vi "Begin.vi"(11 "Image Size":T1=enum."160x120") -> (0 "error out":errorcluster)   [LabVIEW 2011]
doc: "Called before other user functions, this VI is expected to open initial I/O refnums, load in file data, and do all program initialization. Notice that the <B>error out</B> terminal is simply used for data flow. Wiring it to other structures or subVIs ensures that this VI runs first."
uses:
  <vilib>/Rock Robotics/WPI/Camera/WPI_CameraImageSize.ctl
  <vilib>/Rock Robotics/WPI/Joystick/WPI_JoystickDeviceEnum.ctl
  <vilib>/Rock Robotics/WPI/Camera/WPI_CameraWhite Balance Values.ctl
  <vilib>/Rock Robotics/WPI/Camera/WPI_CameraExposure Values.ctl
  <vilib>/Rock Robotics/WPI/Camera/WPI_CameraFrameRate.ctl
  <vilib>/Rock Robotics/SystemInterfaces/DIO/FPGA_DIOPWMChannel.ctl
  <vilib>/Rock Robotics/WPI/Relay/WPI_RelayDirection.ctl
  <vilib>/Rock Robotics/SystemInterfaces/DIO/FPGA_DIORelayChannel.ctl
  <vilib>/Rock Robotics/SystemInterfaces/Typedef/FPGA_TypedefDigitalModule.ctl
  <vilib>/Rock Robotics/SystemInterfaces/DIO/FPGA_DIOChannel.ctl
  <vilib>/Rock Robotics/WPI/Solenoid/WPI_SolenoidChannel.ctl
  <vilib>/Rock Robotics/WPI/MotorControl/WPI_MotorControlOpen Jaguar.vi
  <vilib>/Rock Robotics/WPI/MotorControl/WPI_MotorControlOpen Victor.vi
  <vilib>/Rock Robotics/WPI/RobotDrive/WPI_RobotDriveOpen4MotorWithJaguar.vi
  <vilib>/Rock Robotics/WPI/Solenoid/WPI_SolenoidOpenDouble.vi
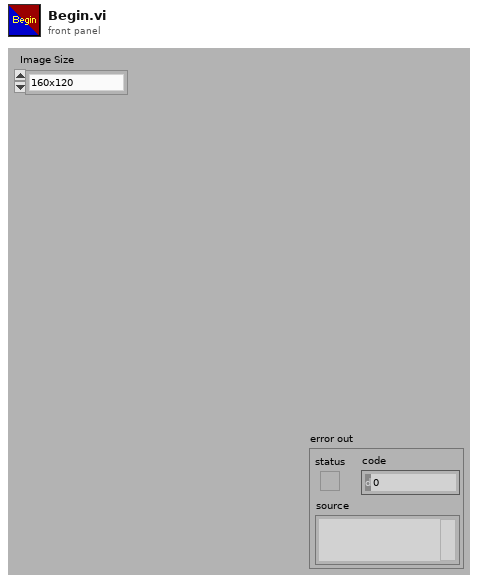
[diagram p1: front panel]
types:
  T1 = typedef "WPI_CameraImageSize.ctl" = enum16{"640x480", "320x240", "160x120"}
  T2 = typedef "WPI_SolenoidChannel.ctl" = enum8{"Solenoid 1", "Solenoid 2", "Solenoid 3", "Solenoid 4", "Solenoid 5", "Solenoid 6", "Solenoid 7", "Solenoid 8", "Invalid"}
  T3 = typedef "FPGA_DIOChannel.ctl" = enum8{"DIO 1", "DIO 2", "DIO 3", "DIO 4", "DIO 5", "DIO 6", "DIO 7", "DIO 8", "DIO 9", "DIO 10", "DIO 11", "DIO 12", "DIO 13", "DIO 14", "Invalid"}
  T4 = typedef "FPGA_TypedefDigitalModule.ctl" = enum16{"Digital Module 1", "Digital Module 2"}
  T5 = typedef "FPGA_DIORelayChannel.ctl" = enum8{"Relay 1", "Relay 2", "Relay 3", "Relay 4", "Relay 5", "Relay 6", "Relay 7", "Relay 8", "Invalid"}
  T6 = typedef "WPI_RelayDirection.ctl" = enum16{"Both directions", "Forward only", "Reverse only"}
  T7 = typedef "FPGA_DIOPWMChannel.ctl" = enum8{"PWM 1", "PWM 2", "PWM 3", "PWM 4", "PWM 5", "PWM 6", "PWM 7", "PWM 8", "PWM 9", "PWM 10", "Invalid"}
  T8 = typedef "WPI_JoystickDeviceEnum.ctl" = enum16{"USB 1", "USB 2", "USB 3", "USB 4", "Kinect 1", "Kinect 2"}
  T9 = typedef "WPI_CameraFrameRate.ctl" = u32
  T10 = typedef "WPI_CameraExposure Values.ctl" = enum16{"Auto", "Flicker-free 50 Hz", "Flicker-free 60 Hz", "Hold current"}
  T11 = typedef "WPI_CameraWhite Balance Values.ctl" = enum16{"Auto", "Fixed indoor", "Fixed outdoor 1", "Fixed outdoor 2", "Fixed fluorescent 1", "Fixed fluorescent 2", "Hold current"}
  T12 = typedef "WPI_MotorControlDeviceRef.ctl" = cluster{"DeviceStatus":errorcluster, "Type":enum16{"PWM", "CAN"}, "PWM":cluster{"Digital Module":T4, "PWM Channel":T7, "DeadBand":T13}, "CAN":cluster{"Device Number":u8, "Control Mode":T14, "Semaphore":T15, "Max Vout":dbl}, "Invert":bool, "TransformRef":T16, "InvTransformRef":T16}
  T13 = typedef "WPI_PWMDeadband.ctl" = cluster{"Name":string, "maxPositivePwm":i32, "minPositivePwm":i32, "centerPwm":i32, "maxNegativePwm":i32, "minNegativePwm":i32, "angularRange":u16}
  T14 = typedef "WPI_CANJaguar_ControlMode.ctl" = enum8{"Percent VBus", "Current", "Speed", "Position", "Voltage"}
  T15 = typedef "Semaphore RefNum" = refnum<k1>
  T16 = typedef "WPI_PWMTransform_ConPane.ctl" = refnum<vi>
  T17 = typedef "WPI_JoystickDevRef.ctl" = cluster{"Device":T8}
  T18 = typedef "WPI_RobotDriveDevRef.ctl" = cluster{"DevStatus":errorcluster, "Motors[]":T12[], "Square Inputs":bool, "Max Output":dbl, "Isochronous":bool}
  T19 = typedef "WPI_RelayDevRef.ctl" = cluster{"DevStatus":errorcluster, "Relay Channel":T5, "Digital Module":T4, "Relay Direction":T6}
  T20 = typedef "WPI_SolenoidDevRef.ctl" = cluster{"DevStatus":errorcluster, "Solenoid Module":T21, "Forward Solenoid Channel":T2, "Reverse Solenoid Channel":T2}
  T21 = typedef "FPGA_TypedefSolenoidModule.ctl" = enum16{"Solenoid Module 1", "Solenoid Module 2"}
  T22 = typedef "WPI_DigitalInputDevRef.ctl" = cluster{"DevStatus":errorcluster, "DIO Channel":T3, "Digital Module":T4}
  T23 = typedef "WPI_CameraDevRef.ctl" = cluster{"Camera Address":string, "CameraStatus":errorcluster, "Acquire Image Notifier":refnum<notifier>}
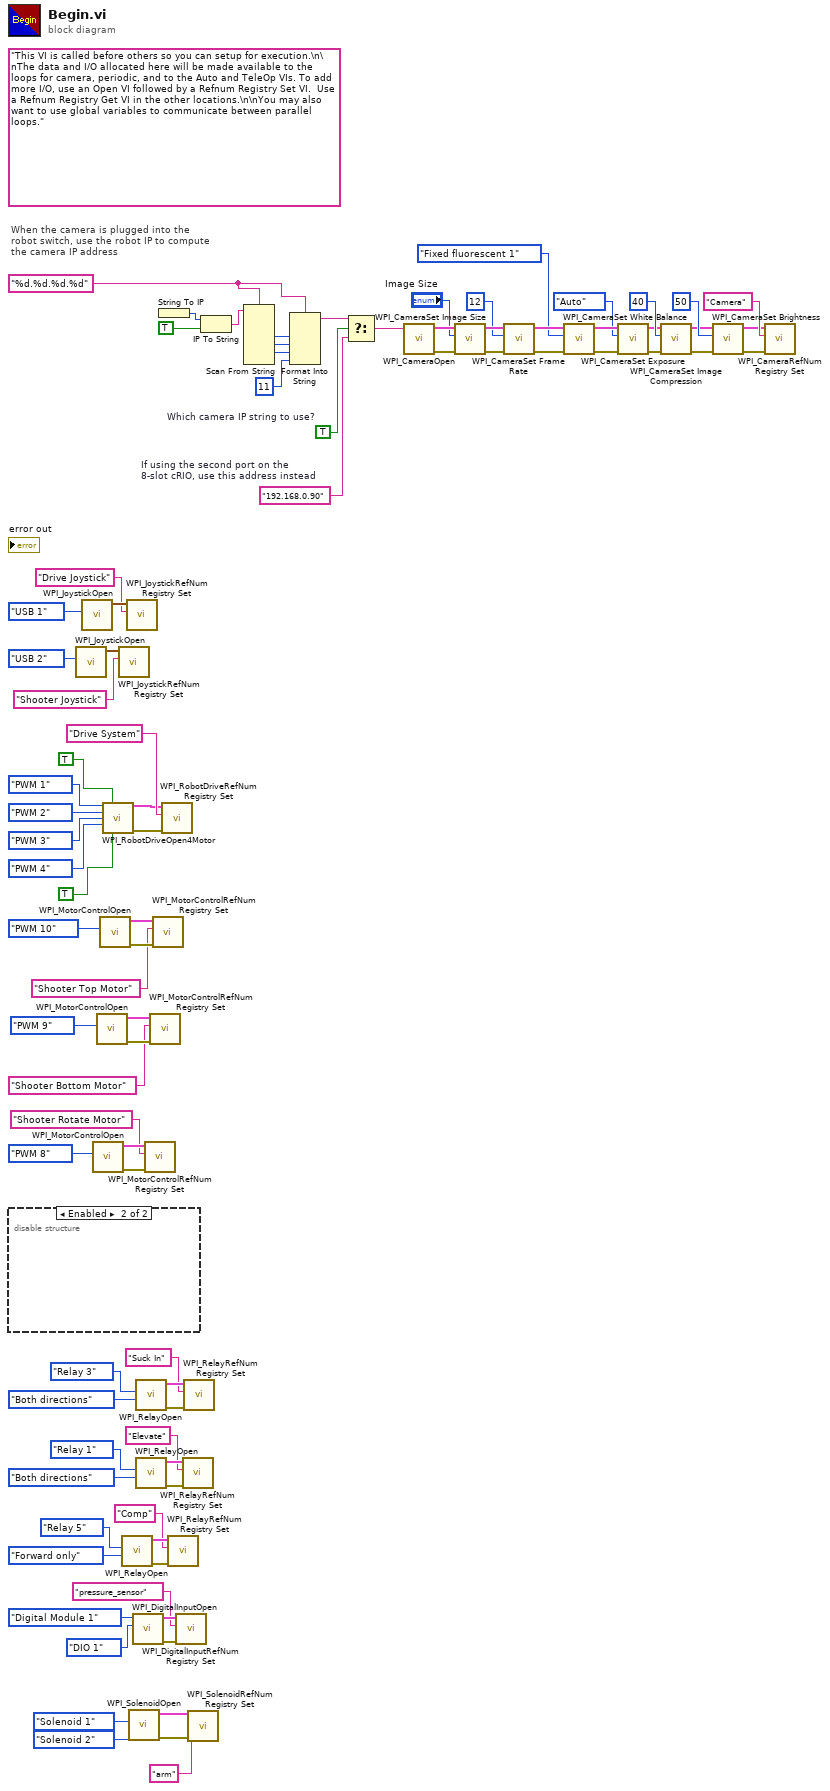
[diagram p0: block diagram]
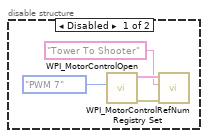
[diagram p2: hidden frame]
diagram:
  w49 = TRUE  # Which camera IP string to use?
  w53 = "%d.%d.%d.%d" ("format string")
  (unwired) "This VI is called before others so you can setup for execution.\n\nThe data and I/O allocated here will be made available to the loops for camera, periodic, and to the Auto and TeleOp VIs. To add more I/O, use an Open VI followed by a Refnum Registry Set VI.  Use a Refnum Registry Get VI in the other locations.\n\nYou may also want to use global variables to communicate between parallel loops."
  w50 = "192.168.0.90"  # If using the second port on the 8-slot cRIO, use this address instead
  # "When the camera is plugged into the\nrobot switch, use the robot IP to compute\nthe camera IP address"
  n1 = disable-structure shown="Enabled" {
    frame Disabled {
      n2 = call-poly <vilib>:"WPI_MotorControlOpen.vi"("PWM Channel"=FPGA_DIOPWMChannel."PWM 7") -> ("error out"=w89:errorcluster, "MotorControlDeviceRef"=w88:T12)  [unwired: 9 in]
      n3 = call <vilib>:"WPI_MotorControlRefNum Registry Set.vi"("error in (no error)"=w89, "refnum name"="Tower To Shooter", "MotorControlDevRef"=w88) -> ()  [unwired: 7 in, 2 out]
    }
    frame Enabled {
    }
  }
  n4 = call <vilib>:"WPI_JoystickOpen.vi"("JoystickDevice"=WPI_JoystickDeviceEnum."USB 2") -> ("JoystickDevRef"=w48:T17)  [unwired: 10 out]
  n5 = call <vilib>:"WPI_JoystickOpen.vi"("JoystickDevice"=WPI_JoystickDeviceEnum."USB 1") -> ("JoystickDevRef"=w83:T17)  [unwired: 10 out]
  n6 = call-poly <vilib>:"WPI_MotorControlOpen.vi"("PWM Channel"=FPGA_DIOPWMChannel."PWM 8") -> ("error out"=w32:errorcluster, "MotorControlDeviceRef"=w31:T12)  [unwired: 9 in]
  n7 = call-poly <vilib>:"WPI_MotorControlOpen.vi"("PWM Channel"=FPGA_DIOPWMChannel."PWM 9") -> ("error out"=w36:errorcluster, "MotorControlDeviceRef"=w35:T12)  [unwired: 9 in]
  n8 = call-poly <vilib>:"WPI_MotorControlOpen.vi"("PWM Channel"=FPGA_DIOPWMChannel."PWM 10") -> ("error out"=w38:errorcluster, "MotorControlDeviceRef"=w37:T12)  [unwired: 9 in]
  n9 = call-poly <vilib>:"WPI_RobotDriveOpen4Motor.vi"("Rear Left Motor"=FPGA_DIOPWMChannel."PWM 1", "Rear Left Motor Inverted"=TRUE, "Rear Right Motor"=FPGA_DIOPWMChannel."PWM 2" ("Rear Left Motor"), "Front Left Motor"=FPGA_DIOPWMChannel."PWM 3" ("Rear Left Motor"), "Front Right Motor"=FPGA_DIOPWMChannel."PWM 4" ("Rear Left Motor"), "Front Left Motor Inverted"=TRUE) -> ("RobotDriveDevRef"=w45:T18, "error out"=w28:errorcluster)  [unwired: 8 in]
  n10 = call <vilib>:"WPI_JoystickRefNum Registry Set.vi"("refnum name"="Shooter Joystick", "JoystickDevRef"=w48) -> ()  [unwired: 1 in, 9 out]
  n11 = call <vilib>:"WPI_RelayOpen.vi"("Relay Direction"=WPI_RelayDirection."Forward only", "Relay Channel"=FPGA_DIORelayChannel."Relay 5") -> ("error out"=w15:errorcluster, "RelayDevRef"=w14:T19)  [unwired: 8 in]
  n12 = call <vilib>:"WPI_JoystickRefNum Registry Set.vi"("refnum name"="Drive Joystick", "JoystickDevRef"=w83) -> ()  [unwired: 1 in, 9 out]
  n13 = call-poly <vilib>:"WPI_SolenoidOpen.vi"("Reverse Solenoid Channel"=WPI_SolenoidChannel."Solenoid 2", "Forward Solenoid Channel"=WPI_SolenoidChannel."Solenoid 1") -> ("error out"=w5:errorcluster, "SolenoidDevRef"=w4:T20)  [unwired: 8 in]
  n14 = call <vilib>:"WPI_DigitalInputOpen.vi"("DIO Channel"=FPGA_DIOChannel."DIO 1", "Digital Module (Module 1)"=FPGA_TypedefDigitalModule."Digital Module 1") -> ("error out"=w8:errorcluster, "DigitalInputDevRef"=w7:T22)  [unwired: 8 in]
  n15 = call <vilib>:"WPI_RelayOpen.vi"("Relay Direction"=WPI_RelayDirection."Both directions", "Relay Channel"=FPGA_DIORelayChannel."Relay 3") -> ("error out"=w23:errorcluster, "RelayDevRef"=w22:T19)  [unwired: 8 in]
  n16 = call <vilib>:"WPI_RelayOpen.vi"("Relay Direction"=WPI_RelayDirection."Both directions", "Relay Channel"=FPGA_DIORelayChannel."Relay 1") -> ("error out"=w21:errorcluster, "RelayDevRef"=w20:T19)  [unwired: 8 in]
  n17 = call <vilib>:"WPI_MotorControlRefNum Registry Set.vi"("error in (no error)"=w32, "refnum name"="Shooter Rotate Motor", "MotorControlDevRef"=w31) -> ()  [unwired: 7 in, 2 out]
  n18 = call <vilib>:"WPI_MotorControlRefNum Registry Set.vi"("error in (no error)"=w36, "refnum name"="Shooter Bottom Motor", "MotorControlDevRef"=w35) -> ()  [unwired: 7 in, 2 out]
  n19 = call <vilib>:"WPI_MotorControlRefNum Registry Set.vi"("error in (no error)"=w38, "refnum name"="Shooter Top Motor", "MotorControlDevRef"=w37) -> ()  [unwired: 7 in, 2 out]
  n20 = String To IP() -> (0:w60:u32)  [unwired: 1 in]
  n21 = call <vilib>:"WPI_RobotDriveRefNum Registry Set.vi"("error in (no error)"=w28, "refnum name"="Drive System", "RobotDriveDevRef"=w45) -> ()  [unwired: 9 out]
  n22 = call <vilib>:"WPI_RelayRefNum Registry Set.vi"("error in (no error)"=w15, "refnum name"="Comp", "RelayDevRef"=w14) -> ()  [unwired: 7 in, 2 out]
  n23 = call <vilib>:"WPI_DigitalInputRefNum Registry Set.vi"("error in (no error)"=w8, "refnum name"="pressure_sensor", "DigitalInputDevRef"=w7) -> ()  [unwired: 7 in, 2 out]
  n24 = call <vilib>:"WPI_RelayRefNum Registry Set.vi"("error in (no error)"=w21, "refnum name"="Elevate", "RelayDevRef"=w20) -> ()  [unwired: 7 in, 2 out]
  n25 = call <vilib>:"WPI_RelayRefNum Registry Set.vi"("error in (no error)"=w23, "refnum name"="Suck In", "RelayDevRef"=w22) -> ()  [unwired: 7 in, 2 out]
  n26 = call <vilib>:"WPI_SolenoidRefNum Registry Set.vi"("error in (no error)"=w5, "refnum name"="arm", "SolenoidDevRef"=w4) -> ()  [unwired: 7 in, 2 out]
  n27 = IP To String(1:TRUE ("dot notation? (F)"), 2:w60) -> (0:w58:string)
  n28 = Scan From String(format string=w53, input string=w58) -> (output 1=w57:i32, output 2=w56:i32, output 3=w55:i32)  [unwired: 7 in, 3 out]
  n29 = Format Into String(format string=w53, w57, w56, w55, 11 ("Compression")) -> (resulting string=w51:string)  [unwired: 2 in, 1 out]
  n30 = Select(t=w51, s=w49, f=w50) -> (s? t:f=w52:string)
  n31 = call <vilib>:"WPI_CameraOpen.vi"("Camera Address"=w52) -> ("error out"=w73:errorcluster, "CameraDevRef"=w74:T23)  [unwired: 1 in, 8 out]
  n32 = call <vilib>:"WPI_CameraSet Image Size.vi"("error in (no error)"=w73, "Image Size"="Image Size", "CameraDevRef"=w74) -> ("error out"=w72:errorcluster, "CameraDevRef Out"=w75:T23)  [unwired: 7 out]
  n33 = call <vilib>:"WPI_CameraSet Frame Rate.vi"("error in (no error)"=w72, "Frame Rate (fps)"=T9 12, "CameraDevRef"=w75) -> ("error out"=w71:errorcluster, "CameraDevRef Out"=w77:T23)  [unwired: 7 out]
  n34 = call <vilib>:"WPI_CameraSet White Balance.vi"("error in (no error)"=w71, "White Balance"=WPI_CameraWhite_Balance_Values."Fixed fluorescent 1", "CameraDevRef"=w77) -> ("error out"=w70:errorcluster, "CameraDevRef Out"=w76:T23)  [unwired: 7 out]
  n35 = call <vilib>:"WPI_CameraSet Exposure.vi"("error in (no error)"=w70, "Exposure"=WPI_CameraExposure_Values."Auto", "CameraDevRef"=w76) -> ("error out"=w69:errorcluster, "CameraDevRef Out"=w79:T23)  [unwired: 7 out]
  n36 = call <vilib>:"WPI_CameraSet Image Compression.vi"("error in (no error)"=w69, "Compression"=40, "CameraDevRef"=w79) -> ("error out"=w68:errorcluster, "CameraDevRef Out"=w78:T23)  [unwired: 7 out]
  n37 = call <vilib>:"WPI_CameraSet Brightness.vi"("error in (no error)"=w68, "Brightness"=50, "CameraDevRef"=w78) -> ("error out"=w66:errorcluster, "CameraDevRef Out"=w67:T23)  [unwired: 7 out]
  n38 = call <vilib>:"WPI_CameraRefNum Registry Set.vi"("error in (no error)"=w66, "refnum name"="Camera", "CameraDevRef"=w67) -> ()  [unwired: 9 out]
